vi "Stop Measurement.vi"(8 "error in (no error)":errorcluster, 10 "Measurement name":string, 11 "Common Measurements in":refnum<class "Common Measurements.lvclass">) -> (0 "error out":errorcluster, 3 "Common Measurements out":refnum<class "Common Measurements.lvclass">)   [LabVIEW 2015, in "Common Measurements.lvclass"]
uses:
  Common Measurements.lvclass
  Common Measurements.lvclass/Common Measurements.ctl
  Mag Lab Measure Controller/Mag Lab Measure Controller.lvclass
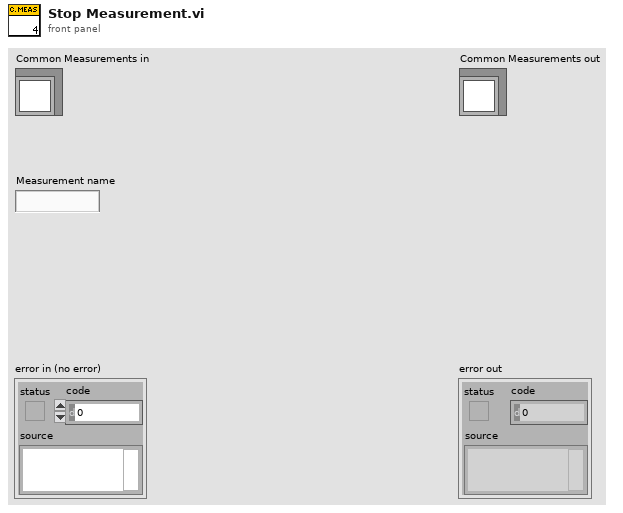
[diagram p1: front panel]
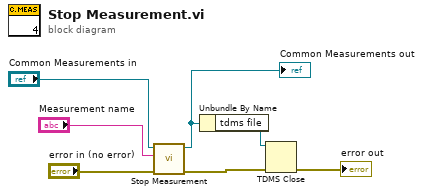
[diagram p0: block diagram]
diagram:
  n1 = call-parent "Stop Measurement.vi"("error in (no error)"="error in (no error)", "Measurement name"="Measurement name", "Mag Lab Measure Controller in"="Common Measurements in") -> ("error out"=w7:errorcluster, "Mag Lab Measure Controller out"=w2:refnum<class "Common Measurements.lvclass">)  [unwired: 7 in]
  "Common Measurements out" <- w2
  n2 = Unbundle By Name(w2) -> ("tdms file"=w1:refnum<k34>)
  n3 = TDMS Close(8:w7, 11:w1) -> (0:→"error out":errorcluster)  [unwired: 1 out]
